vi "host.vi"() -> ()   [LabVIEW 2020]
uses:
  b4957acc-33c7-4f51-b6c8-be02e890b770.vi
  <vilib>/Array/Sort 2D Array - Pop Stack.vi
  <vilib>/Array/Sort 2D Array - Push Stack.vi
  b4957acc-33c7-4f51-b6c8-be02e890b770.vi/269d4b3b-47f5-49e3-8884-44851e4dd9d5.vi
  b4957acc-33c7-4f51-b6c8-be02e890b770.vi/6d99389c-673d-4efb-bf33-19b32bcf4cf8.vi
  <vilib>/FPGAPlugInAG/cRIO-9035/niLvFpga_Open_cRIO-9035.vi
  <vilib>/FPGAPlugInAG/cRIO-9035/niLvFpga_Reset_cRIO-9035.vi
  <vilib>/Utility/error.llb/Error Cluster From Error Code.vi
  <vilib>/rvi/errors/niLvFpgaAdjustHostInterfaceError.vi
  <vilib>/FPGAPlugInAG/cRIO-9035/niLvFpga_Run_cRIO-9035.vi
  <vilib>/FPGAPlugInAG/cRIO-9035/niLvFpga_Close_cRIO-9035.vi
  <vilib>/rvi/interface/nirviOpenFPGA/nirviOpenFPGA.xnode
  FPGA Bitfiles/project_FPGATarget_target_C55-F1LgfNE.lvbitx
  target.vi
  <vilib>/rvi/interface/nirviMethod/nirviMethod.xnode
  <vilib>/rvi/interface/nirviReadWriteControl/nirviReadWriteControl.xnode
  <vilib>/rvi/interface/nirviCloseFPGA/nirviCloseFPGA.xnode
  <vilib>/Analysis/NI_AALBase.lvlib
  <vilib>/FPGAPlugInAG/cRIO-9035/niLvFpga_StartFifo_cRIO-9035.vi
  <vilib>/rvi/errors/niLvFpgaMergeErrorWithErrorCode.vi
  <vilib>/FPGAPlugInAG/cRIO-9035/niLvFpga_WriteFifo_cRIO-9035.vi
  NiFpgaLv.dll
  <vilib>/FPGAPlugInAG/cRIO-9035/niLvFpga_ReadFifo_cRIO-9035.vi
panel:
  out "Data":sgl[](array[numeric])
  out "error out":errorcluster
  out "Timed Out? FIFO out REAL":bool
  out "Timed Out? FIFO in REAL":bool
  out "sorted 2D array":sgl[][](array[numeric])
  out "input data":sgl[](graph)
  out "sort time (ms)":dbl
  out "Elements Remaining":u32
  out "Real sorted signal":sgl[](graph)
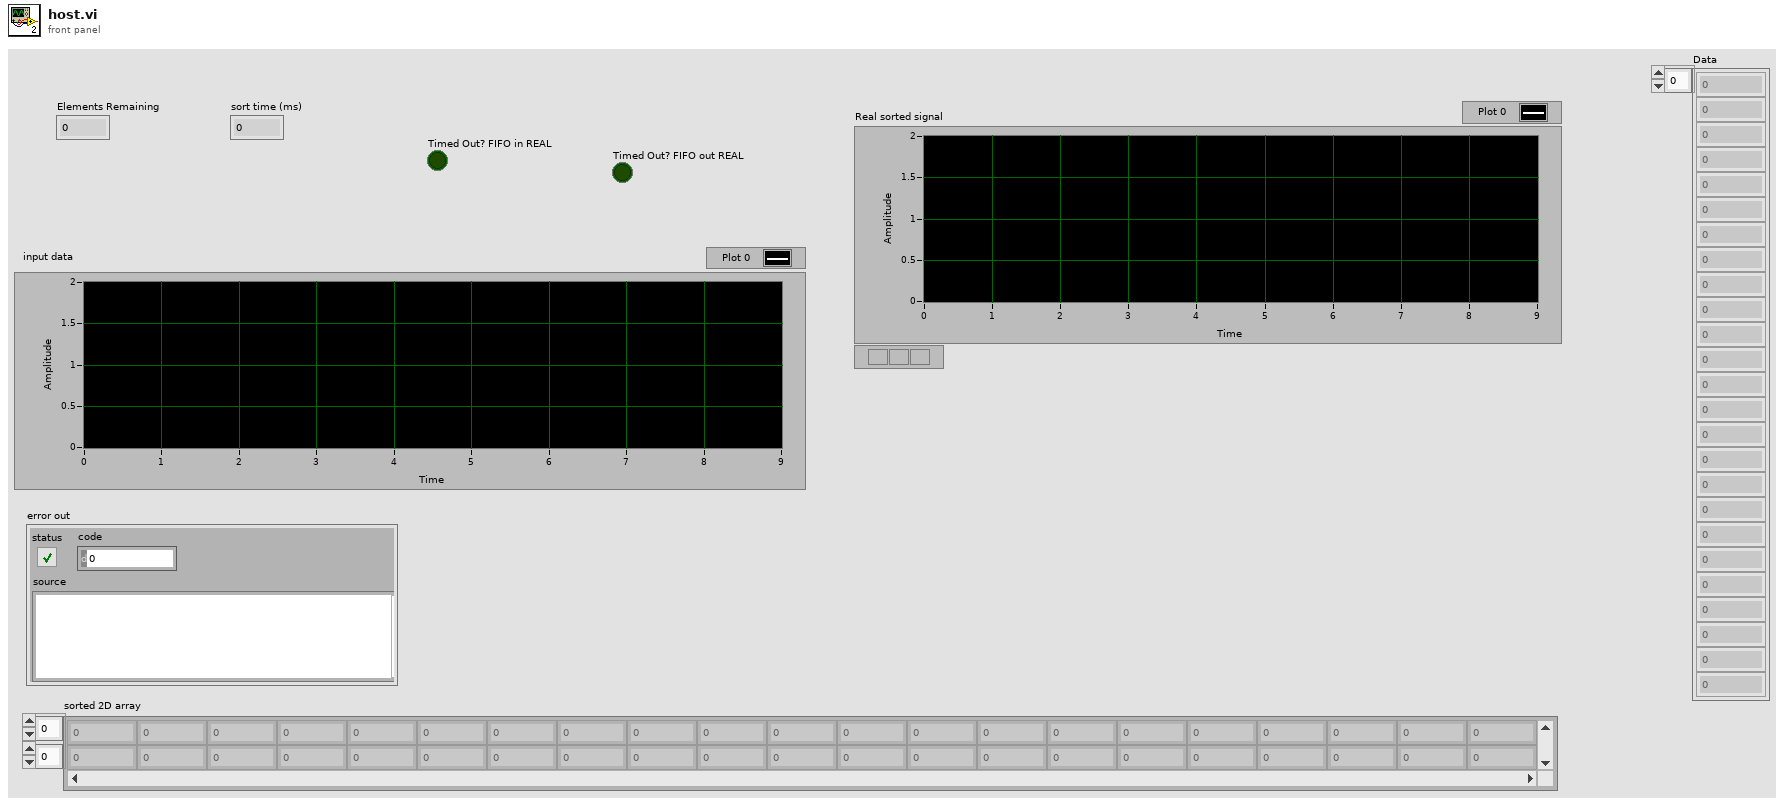
[diagram p1: front panel]
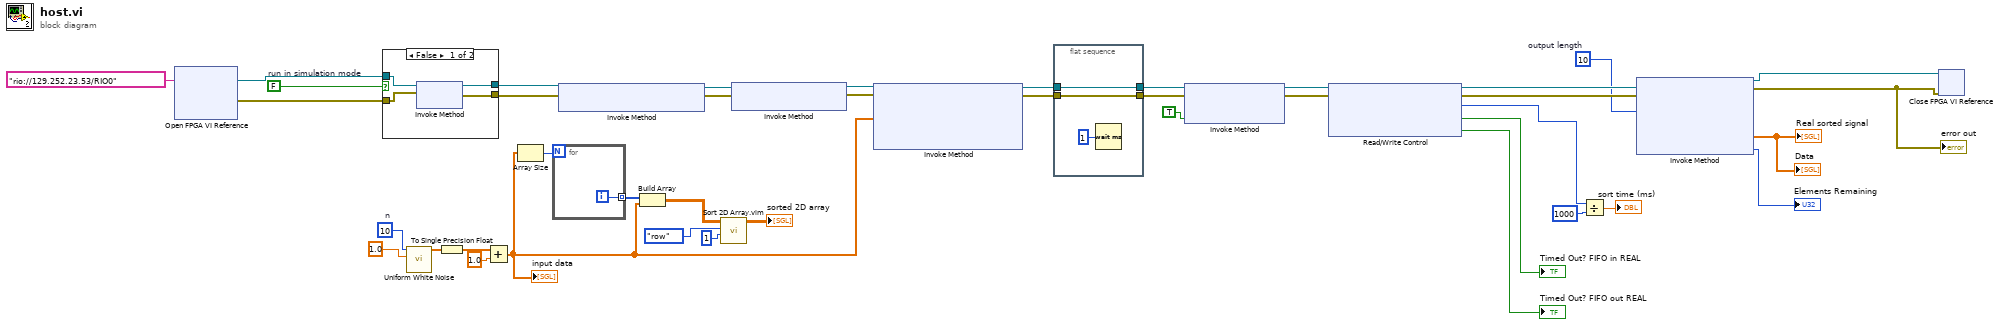
[diagram p0: block diagram]
diagram:
  w9 = FALSE  # run in simulation mode
  w23 = 10  # n
  w16 = u32 10  # output length
  n1 = xnode "Open FPGA VI Reference"("resource name"=tag "rio://129.252.23.53/RIO0") -> ("FPGA VI Reference Out"=w8:refnum<k20>, "error out"=w7:errorcluster)  [unwired: 1 in]
  n2 = case shown="False" w9 {
    tunnel: w8 -> [w45 w46]
    tunnel: w7 -> [w44 w47]
    tunnel: [w43 w46] -> w6
    tunnel: [w42 w47] -> w5
    frame False {
      n3 = xnode "Invoke Method"("FPGA VI Reference In"=w45, "error in"=w44) -> ("FPGA VI Reference Out"=w43:refnum<k20>, "error out"=w42:errorcluster)
    }
    frame True {
    }
  }
  n4 = call <vilib>:"Uniform White Noise.vi"("amplitude"=1.0, "samples"=w23) -> ("uniform white noise"=w22:dbl[])  [unwired: 8 in, 1 out]
  n5 = To Single Precision Float(number=w22) -> (single precision float=w21:sgl[])
  n6 = Add(x=w21, y=sgl 1.0 ("amplitude")) -> (x+y=w4:sgl[])
  "input data" <- w4
  n7 = Array Size(array=w4) -> (size(s)=w28:i32)
  n8 = for {
    N: w28 -> [_]
    tunnel: [w48] -> w27 mode=indexing
    i -> [w48]
  }
  n9 = xnode "Invoke Method"("FPGA VI Reference In"=w6, "error in"=w5) -> ("FPGA VI Reference Out"=w20:refnum<k20>, "error out"=w19:errorcluster)
  n10 = Build Array(w27, w4) -> (w26:sgl[][])
  n11 = call "Sort 2D Array.vim"("index"=1, "dimension to index (column)"=enum16{"column", "row"}."row", "2D array"=w26) -> ("sorted 2D array"=→"sorted 2D array":sgl[][])  [unwired: 7 in, 1 out]
  n12 = xnode "Invoke Method"("FPGA VI Reference In"=w20, "error in"=w19) -> ("FPGA VI Reference Out"=w14:refnum<k20>, "error out"=w15:errorcluster)
  n13 = xnode "Invoke Method"("FPGA VI Reference In"=w14, "error in"=w15, "Data"=w4) -> ("FPGA VI Reference Out"=w18:refnum<k20>, "error out"=w17:errorcluster)  [unwired: 1 in, 1 out]
  n14 = flat-sequence {
    tunnel: [w50] -> w11
    tunnel: w18 -> [w50]
    tunnel: [w49] -> w10
    tunnel: w17 -> [w49]
    frame #0 {
      n15 = Wait (ms)(milliseconds to wait=u32 1) -> ()  [unwired: 1 out]
    }
  }
  n16 = xnode "Invoke Method"("FPGA VI Reference In"=w11, "error in"=w10, "Wait Until Done (F)"=TRUE) -> ("FPGA VI Reference Out"=w38:refnum<k20>, "error out"=w37:errorcluster)
  n17 = xnode "Read/Write Control"("FPGA VI Reference In"=w38, "error in"=w37) -> ("FPGA VI Reference Out"=w32:refnum<k20>, "error out"=w31:errorcluster, "sort time (us)"=w36:u32, "Timed Out? FIFO in REAL"=→"Timed Out? FIFO in REAL":bool, "Timed Out? FIFO out REAL"=→"Timed Out? FIFO out REAL":bool)
  n18 = Divide(x=w36, y=u32 1000) -> (x/y=→"sort time (ms)":dbl)
  n19 = xnode "Invoke Method"("FPGA VI Reference In"=w32, "error in"=w31, "Number of Elements"=w16) -> ("FPGA VI Reference Out"=w2:refnum<k20>, "error out"=w1:errorcluster, "Data"=→"Real sorted signal" →"Data":sgl[], "Elements Remaining"=→"Elements Remaining":u32)  [unwired: 1 in]
  "error out" <- w1
  n20 = xnode "Close FPGA VI Reference"("FPGA VI Reference In"=w2, "error in"=w1) -> ()  [unwired: 1 out]
